vi "Table to JSON Schema.vi"(8 "error in (no error)":errorcluster, 10 "Table":string[][](table), 11 "JSON Schema in":string) -> (0 "error out":errorcluster, 3 "JSON Schema out":string)   [LabVIEW 2019, in "JSON-Schema.lvlib"]
doc: "<b>InfoTable</b> is a table.\n- First row: name, description, units, (min_value, min_value)\n- Remainder: values"
uses:
  JSON-Schema.lvlib
  92616eff-9b0c-4e28-944c-aab5ae23ad69.vi
  <vilib>/JDP Science/JSONtext/Next JSON Value.vi
  <vilib>/JDP Science/JSONtext/String Subset.vi
  <vilib>/JDP Science/JSONtext/Parsing/Advance past next JSON Value (inlined COPY).vi
  <vilib>/JDP Science/JSONtext/Parsing/Advance past whitespace.vi
  <vilib>/JDP Science/JSONtext/Parsing/Advance past String.vi
  <vilib>/JDP Science/JSONtext/Parsing/Advance past Number.vi
  <vilib>/JDP Science/JSONtext/Parsing/Advance past Line Ending.vi
  <vilib>/JDP Science/JSONtext/Parsing/Parse Full Path or Item Name.vi
  <vilib>/JDP Science/JSONtext/Parsing/Advance past Array.vi
  <vilib>/JDP Science/JSONtext/Parsing/Advance past Object.vi
  <vilib>/JDP Science/JSONtext/support/Error Cluster From Code.vi
  <vilib>/JDP Science/JSONtext/Offset/Find Item Locations by Path.vi
  <vilib>/JDP Science/JSONtext/Variant to JSON Text.vi
  <vilib>/JDP Science/JSONtext/LVClass Serializer/JSONtext LVClass Serializer.lvclass
  <vilib>/JDP Science/JSONtext/JSONtext.lvlib
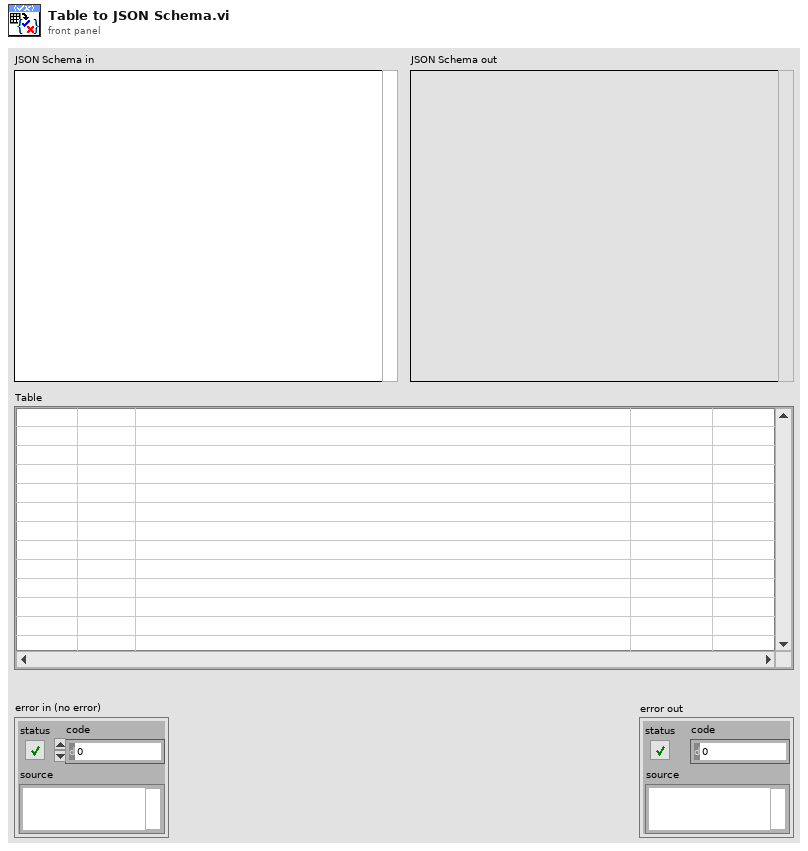
[diagram p1: front panel]
types:
  T1 = typedef "JSONtext.lvlib/JSON Value Type.ctl" = enum16{"Not a JSON Value", "JSON Object", "JSON Array", "String", "Number", "true", "false", "null"}
  T2 = enum32{"Bad", "Idle", "Run top level", "Running"}
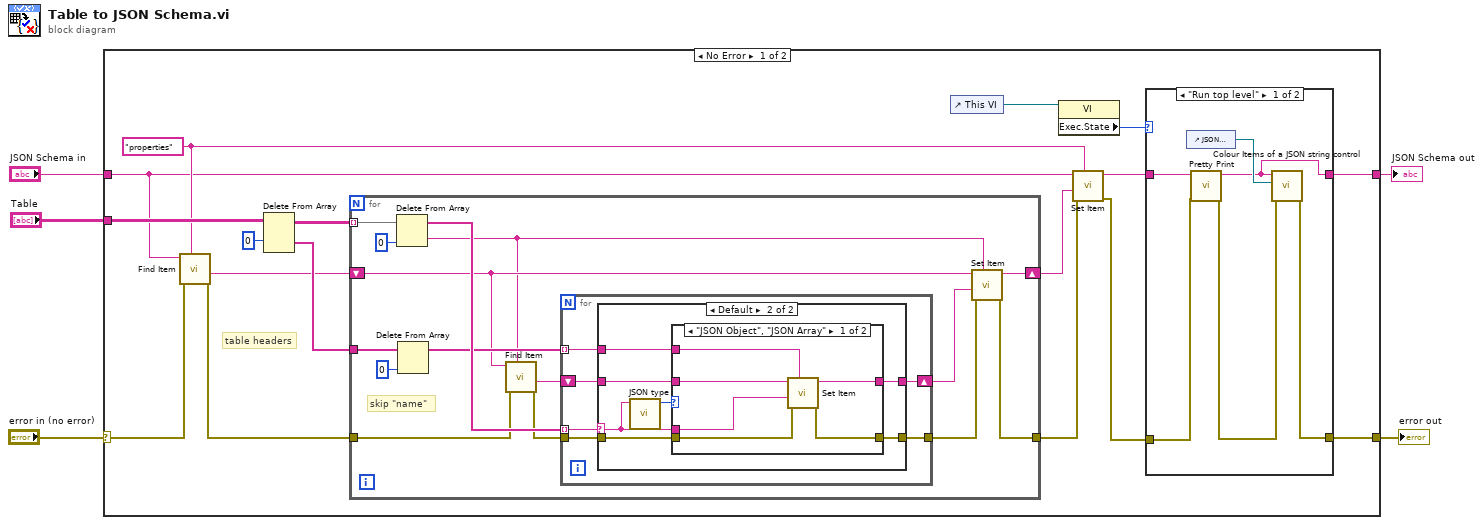
[diagram p0: block diagram]
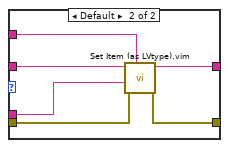
[diagram p4: hidden frame]
diagram:
  n1 = case shown="No Error" "error in (no error)" {
    selector: "error in (no error)" -> [w17 w73]
    tunnel: "Table" -> [w22 _]
    tunnel: [w7 w73] -> w3
    tunnel: "JSON Schema in" -> [w12 _]
    tunnel: [w6 _] -> w1
    frame No Error {
      w15 = "properties" ("$Path or Item Name")
      # "table headers"
      n2 = call <vilib>:"Find Item.vi"("$Path or Item Name"=w15, "error in (no error)"=w17, "JSON"=w12) -> ("error out"=w16:errorcluster, "<JSON>"=w18:string)  [unwired: 5 in, 2 out]
      n3 = Delete From Array(array=w22, index (row)=0) -> (deleted portion=w19:string[], array with subset deleted=w21:string[][])  [unwired: 2 in]
      n4 = for {
        tunnel: w21 -> [w45] mode=indexing
        shift-right: [w42] -> w14
        shift-left: w18 -> [w35]
        tunnel: w19 -> [w39]
        tunnel: [w40] -> w13
        tunnel: w16 -> [w31]
        # "skip \"name\""
        n5 = Delete From Array(array=w45, index=0) -> (deleted portion=w34:string, array with subset deleted=w44:string[])  [unwired: 1 in]
        n6 = Delete From Array(array=w39, index=0) -> (array with subset deleted=w36:string[])  [unwired: 1 in, 1 out]
        n7 = call <vilib>:"Find Item.vi"("$Path or Item Name"=w34, "error in (no error)"=w31, "JSON"=w35) -> ("error out"=w32:errorcluster, "<JSON>"=w33:string)  [unwired: 5 in, 2 out]
        n8 = for {
          tunnel: w44 -> [w46] mode=indexing
          tunnel: w36 -> [w47] mode=indexing
          shift-right: [w50] -> w43
          shift-left: w33 -> [w51]
          tunnel: [w49] -> w41
          tunnel: w32 -> [w48]
          n9 = case shown="Default" w46 {
            selector: w46 -> [_ w54]
            tunnel: w51 -> [w53 w60]
            tunnel: [w53 w59] -> w50
            tunnel: [w52 w58] -> w49
            tunnel: w48 -> [w52 w57]
            tunnel: w47 -> [_ w56]
            frame "" {
            }
            frame Default {
              n10 = call <vilib>:"JSON type.vi"("JSON"=w54) -> ("JSON Value Type"=w55:T1)  [unwired: 9 in, 1 out]
              n11 = case shown="\"JSON Object\", \"JSON Array\"" w55 {
                tunnel: w60 -> [w66 w69]
                tunnel: [w65 w70] -> w59
                tunnel: [w61 w67] -> w58
                tunnel: w57 -> [w62 w68]
                tunnel: w56 -> [w64 w72]
                tunnel: w54 -> [w63 w71]
                frame "JSON Object", "JSON Array" {
                  n12 = call <vilib>:"Set Item.vi"("$Path or Item Name"=w64, "error in (no error)"=w62, "JSON to Insert"=w63, "JSON"=w66) -> ("error out"=w61:errorcluster, "<JSON>"=w65:string)  [unwired: 4 in, 1 out]
                }
                frame Default {
                  n13 = call "Set Item (as LVtype).vim"("$Path or Item Name"=w72, "error in (no error)"=w68, "Anything"=w71, "JSON"=w69) -> ("error out"=w67:errorcluster, "<JSON>"=w70:string)  [unwired: 4 in, 1 out]
                }
              }
            }
          }
        }
        n14 = call <vilib>:"Set Item.vi"("$Path or Item Name"=w34, "error in (no error)"=w41, "JSON to Insert"=w43, "JSON"=w35) -> ("error out"=w40:errorcluster, "<JSON>"=w42:string)  [unwired: 4 in, 1 out]
      }
      n15 = control-ref of="This VI"() -> (w11:refnum<vi>)
      n16 = property class="VI"(reference=w11) -> ("Exec.State"=w10:T2)  [unwired: 1 in, 2 out]
      n17 = call <vilib>:"Set Item.vi"("$Path or Item Name"=w15, "error in (no error)"=w13, "JSON to Insert"=w14, "JSON"=w12) -> ("error out"=w9:errorcluster, "<JSON>"=w8:string)  [unwired: 4 in, 1 out]
      n18 = case shown="\"Run top level\"" w10 {
        tunnel: w9 -> [w27 w29]
        tunnel: w8 -> [w26 w30]
        tunnel: [w25 w29] -> w7
        tunnel: [w23 w30] -> w6
        frame "Run top level" {
          n19 = control-ref of="JSON Schema out"() -> (w28:refnum<vi>)
          n20 = call <vilib>:"Pretty Print.vi"("error in (no error)"=w27, "JSON"=w26) -> ("error out"=w24:errorcluster, "<JSON>"=w23:string)  [unwired: 7 in, 1 out]
          n21 = call <vilib>:"Colour Items of a JSON string control.vi"("error in (no error)"=w24, "String Control"=w28, "JSON"=w23) -> ("error out"=w25:errorcluster)  [unwired: 8 in]
        }
        frame Default {
        }
      }
    }
    frame Error {
    }
  }
  "JSON Schema out" <- w1
  "error out" <- w3
